vi "get_broken_vi_log.vi"(8 "error in":errorcluster) -> (0 "error out":errorcluster, 3 "broken vi log":string)   [LabVIEW 2021]
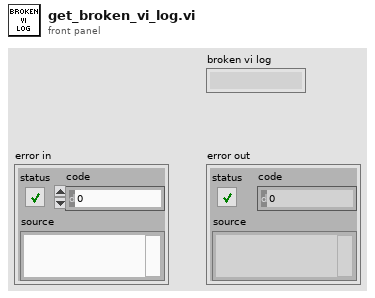
[diagram p1: front panel]
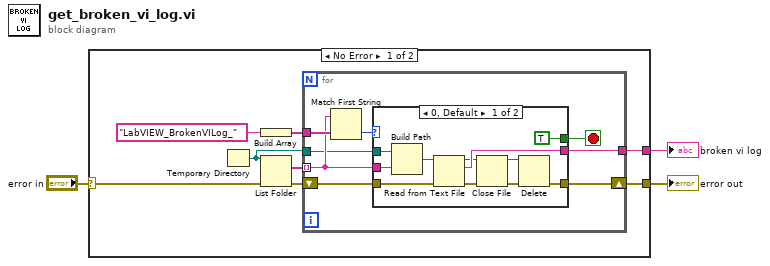
[diagram p0: block diagram]
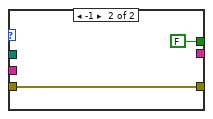
[diagram p2: hidden frame]
diagram:
  n1 = case shown="No Error" "error in" {
    selector: "error in" -> [w6 w33]
    tunnel: [w5 w33] -> w2
    tunnel: [w4 _] -> w1
    frame No Error {
      n2 = Temporary Directory() -> (w8:path)
      n3 = Build Array("LabVIEW_BrokenVILog_" ("string")) -> (w9:string[])
      n4 = List Folder(path=w8, error in=w6) -> (filenames=w11:string[], error out=w7:errorcluster)  [unwired: 2 in, 2 out]
      n5 = for {
        tunnel: w11 -> [w16] mode=indexing
        tunnel: w9 -> [w19]
        tunnel: w8 -> [w15]
        shift-right: [w13] -> w5
        shift-left: w7 -> [w14]
        tunnel: [w12] -> w4
        stop <- w17 stop-if-true
        n6 = Match First String(2:w19, 3:w16) -> (0:w18:i32)  [unwired: 1 out]
        n7 = case shown="0, Default" w18 {
          tunnel: [TRUE FALSE] -> w17
          tunnel: w16 -> [w28 _]
          tunnel: w15 -> [w29 _]
          tunnel: w14 -> [w26 w31]
          tunnel: [w24 w31] -> w13
          tunnel: [w25 _] -> w12
          frame 0, Default {
            n8 = Build Path(base path=w29, name or relative path=w28) -> (appended path=w27:path)
            n9 = Read from Text File(file (use dialog)=w27, error in=w26) -> (refnum out=w22:refnum<file>, text=w25:string, error out=w23:errorcluster)  [unwired: 2 in, 1 out]
            n10 = Close File(refnum=w22, error in=w23) -> (path=w20:path, error out=w21:errorcluster)
            n11 = Delete(path (use dialog)=w20, error in=w21) -> (error out=w24:errorcluster)  [unwired: 3 in, 2 out]
          }
          frame -1 {
          }
        }
      }
    }
    frame Error {
    }
  }
  "error out" <- w2
  "broken vi log" <- w1
